vi "VariantToProperties.vi"(8 "error in (no error)":errorcluster, 11 "ChromaPowerSupplyModel in":refnum<class "ChromaPowerSupplyModel.lvclass">) -> (0 "error out":errorcluster, 1 "Measurements":T2, 2 "Device Settings":T3 caption="Device(s)Settings", 3 "ChromaPowerSupplyModel out":refnum<class "ChromaPowerSupplyModel.lvclass">, 4 "Measurement Refresh Time (ms)":u32, 6 "Database Settings":T1)   [LabVIEW 2018, in "AcPwrPlugins.lvlib" / "ChromaPowerSupplyModel.lvclass"]
uses:
  ChromaPowerSupplyModel.lvclass
  C:/Projects/SmartGrid/ICDAS/NistPluggableModules/AcPwr/AcPwrPlugins/AcPwrBaseClass/AcPwrBase.lvclass
  ChromaPowerSupplyClass/TypeDefs/Device(s)Settings.ctl
  ChromaPowerSupplyClass/TypeDefs/Measurements.ctl
  TypeDefs/Database Settings.ctl
  AcPwrBaseClass/AcPwrBase.lvclass/AcPwrBase.ctl
  AcPwrBaseClass/Accessors/Read BaseConfig.vi
  ChromaPowerSupplyClass/ChromaPowerSupply.lvclass
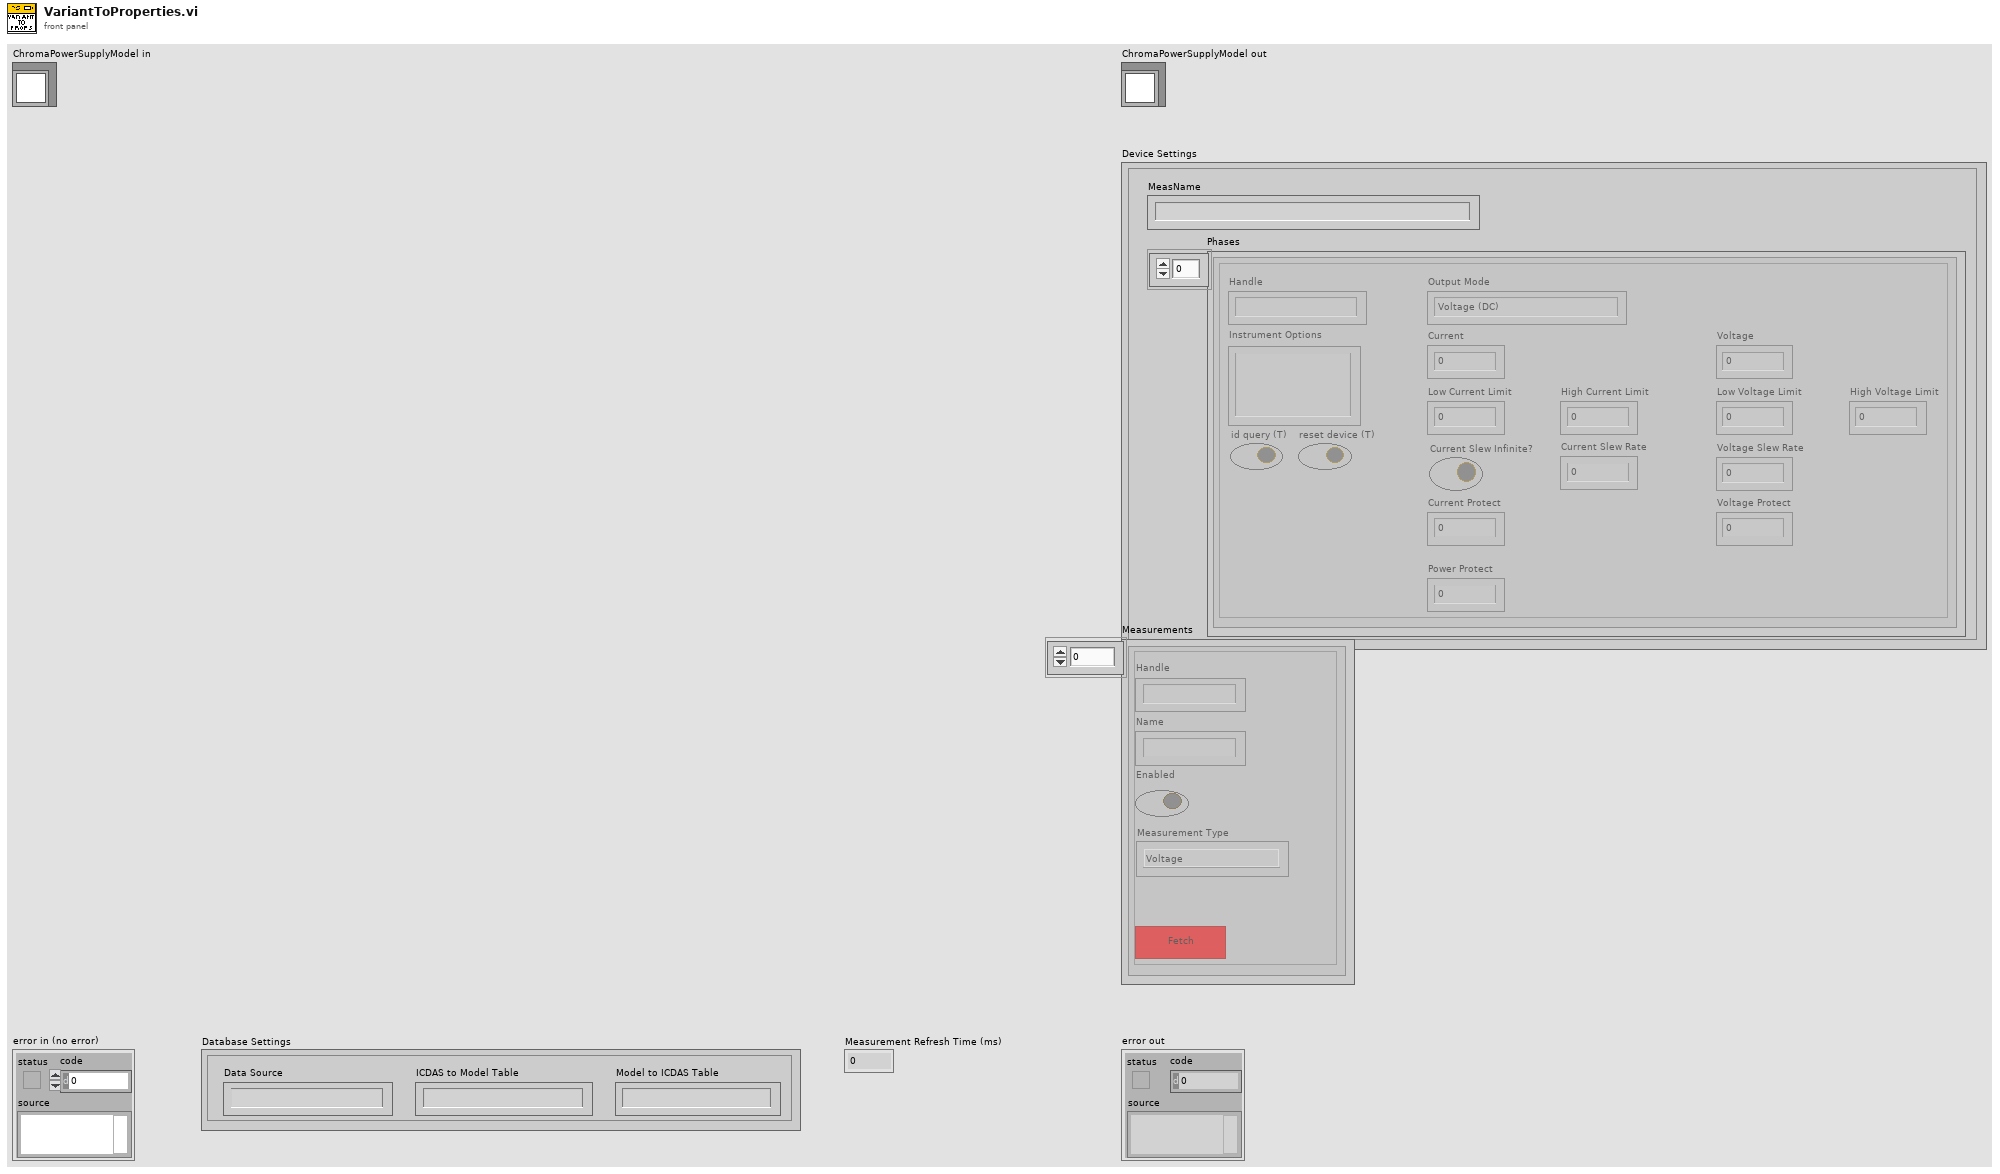
[diagram p1: front panel]
types:
  T1 = typedef "AcPwrPlugins.lvlib/ChromaPowerSupplyModel.lvclass/Database Settings.ctl" = cluster{"Data Source":string, "ICDAS to Model Table":string, "Model to ICDAS Table":string}
  T2 = typedef "AcPwrPlugins.lvlib/ChromaPowerSupply.lvclass/Measurements.ctl" = cluster{"Handle":string, "Name":string, "Enabled":bool, "Measurement Value":dbl, "btnMeasFetch":bool, "ProtectionStatusString":string, "Measurement Type":enum16{"Voltage", "Current", "Power"}}[]
  T3 = typedef "AcPwrPlugins.lvlib/ChromaPowerSupply.lvclass/Device(s)Settings.ctl" = cluster{"Phases":cluster{"Handle":string, "Instrument Options":string, "id query (T)":bool, "reset device (T)":bool, "Timing":cluster{"TimingOn":enum16{""}, "Hours":u32, "Minutes":u32, "Seconds":dbl, "CutoffVoltage":dbl}, "Connected":bool, "Output Mode":enum16{"Voltage (DC)", "Current (DC)"}, "Voltage":dbl, "Current":dbl, "High Voltage Limit":dbl, "High Current Limit":dbl, "Power Protect":dbl, "Current Protect":dbl, "Voltage Protect":dbl, "Low Current Limit":dbl, "Low Voltage Limit":dbl, "Current Slew Rate":dbl, "Voltage Slew Rate":dbl, "Current Slew Infinite?":bool}[], "MeasName":string}
  T4 = typedef "AcPwrPlugins.lvlib/AcPwrBase.lvclass/BaseConfig.ctl" = cluster{"Frequency":dbl, "FrequencyRange":dbl[], "Phases":T5[], "Name":string, "PluginConfigVariant":variant, "PluginMeasVariant":variant}
  T5 = typedef "AcPwrPlugins.lvlib/AcPwrBase.lvclass/Phase.ctl" = cluster{"Name":string, "Enabled":bool, "VoltageLevel":dbl, "Handle":string, "VoltageRange":dbl[], "Connected":bool, "CurrentLimit":dbl, "Waveform":string}
  T6 = cluster{"Device(s)Settings":T3, "Database Settings":T1}
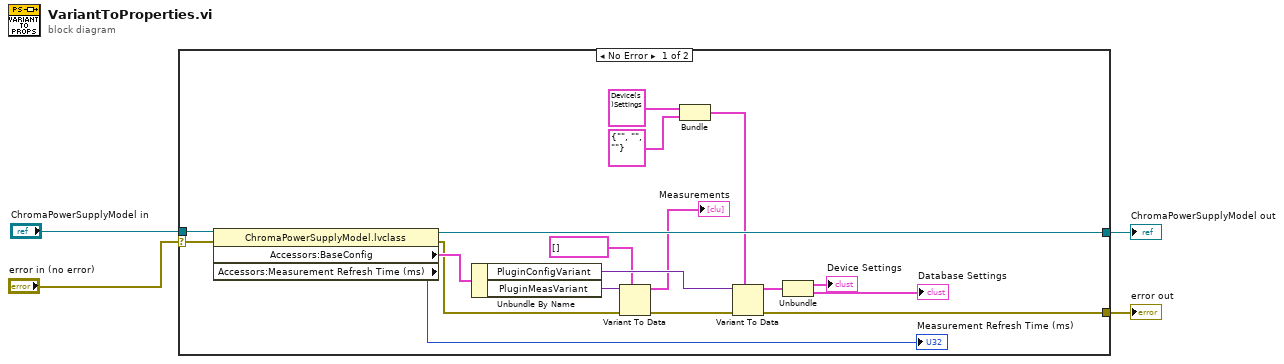
[diagram p0: block diagram]
diagram:
  n1 = case shown="No Error" "error in (no error)" {
    selector: "error in (no error)" -> [w20 w24]
    tunnel: [w22 w24] -> w1
    tunnel: "ChromaPowerSupplyModel in" -> [w21 w23]
    tunnel: [w19 w23] -> w2
    frame No Error {
      n2 = property class="ChromaPowerSupplyModel.lvclass"(reference=w21, error in=w20) -> (reference out=w19:refnum<class "ChromaPowerSupplyModel.lvclass">, error out=w17:errorcluster, "Accessors:BaseConfig"=w18:T4, "Accessors:Measurement Refresh Time (ms)"=→"Measurement Refresh Time (ms)":u32)
      n3 = Unbundle By Name(w18) -> ("PluginConfigVariant"=w14:variant, "PluginMeasVariant"=w16:variant)
      n4 = Variant To Data(error in=w17, type=T2 [] ("Measurements"), Variant=w16) -> (data=→"Measurements":T2, error out=w15:errorcluster)
      n5 = Bundle("Device(s)Settings"=T3 {"Phases"=[{"Handle"="", "Instrument Options"="", "id query (T)"=TRUE, "reset device (T)"=TRUE, "Timing"={"TimingOn"=enum."", "Hours"=0, "Minutes"=0, "Seconds"=0.0, "CutoffVoltage"=0.0}, "Connected"=FALSE, "Output Mode"=enum."Voltage (DC)", "Voltage"=0.0, "Current"=0.0, "High Voltage Limit"=0.0, "High Current Limit"=0.0, "Power Protect"=0.0, "Current Protect"=0.0, "Voltage Protect"=0.0, "Low Current Limit"=0.0, "Low Voltage Limit"=0.0, "Current Slew Rate"=0.0, "Voltage Slew Rate"=0.0, "Current Slew Infinite?"=TRUE}], "MeasName"=""}, "Database Settings"=T1 {"Data Source"="", "ICDAS to Model Table"="", "Model to ICDAS Table"=""}) -> (w10:T6)  [unwired: 1 in]
      n6 = Variant To Data(error in=w15, type=w10, Variant=w14) -> (data=w7:T6, error out=w22:errorcluster)
      n7 = Unbundle(w7) -> ("Device(s)Settings"=→"Device Settings":T3, "Database Settings"=→"Database Settings":T1)
    }
    frame Error {
    }
  }
  "error out" <- w1
  "ChromaPowerSupplyModel out" <- w2
